vi "1.2.1-ParseYPR.vi"(10 "Serial Byte":u8) -> (1 "Yaw":i16, 2 "Heading (out)":T1)   [LabVIEW 2010]
doc: "This VI parses Yaw, Pitch, and Roll (YPR) data from the VectorNav. In response to a YPR Read Request, the VectorNav will reply in the form \"$VNYPR,XX,-XXX.XX,-XXX.XX,+XXX.XX*XX\" (where X is a digit from 0-9). This string is in the form \"$<command type>,<access ID>, <yaw>,<pitch>,<roll>\".\n\nThe VI first waits for a $, then checks to make sure it has read \"VNYPR,\" correctly, then adds up each of the XX values and saves them appropriately. Since it receives these values one byte at a time , it must do some simple fixed point math to make sure the appropriate decimal value is saved."
uses:
  1.2.1-ParseYPR.ctl
panel:
  in  "Heading (in)":T1 {"Yaw" format="%.42g"; "Pitch" format="%.42g"; "Roll" format="%.42g"}
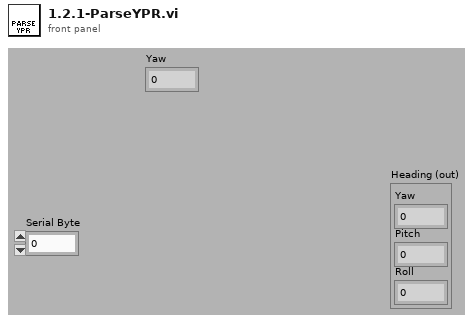
[diagram p1: front panel]
types:
  T1 = cluster{"Yaw":fxp<+/-,64,32>, "Pitch":fxp<+/-,64,32>, "Roll":fxp<+/-,64,32>}
  T2 = typedef "1.2.1-ParseYPR.ctl" = enum16{"Wait for $", "Check VNYPR", "Read numbers"}
  T3 = enum16{"Initialize", "Yaw", "Pitch", "Roll", "Done"}
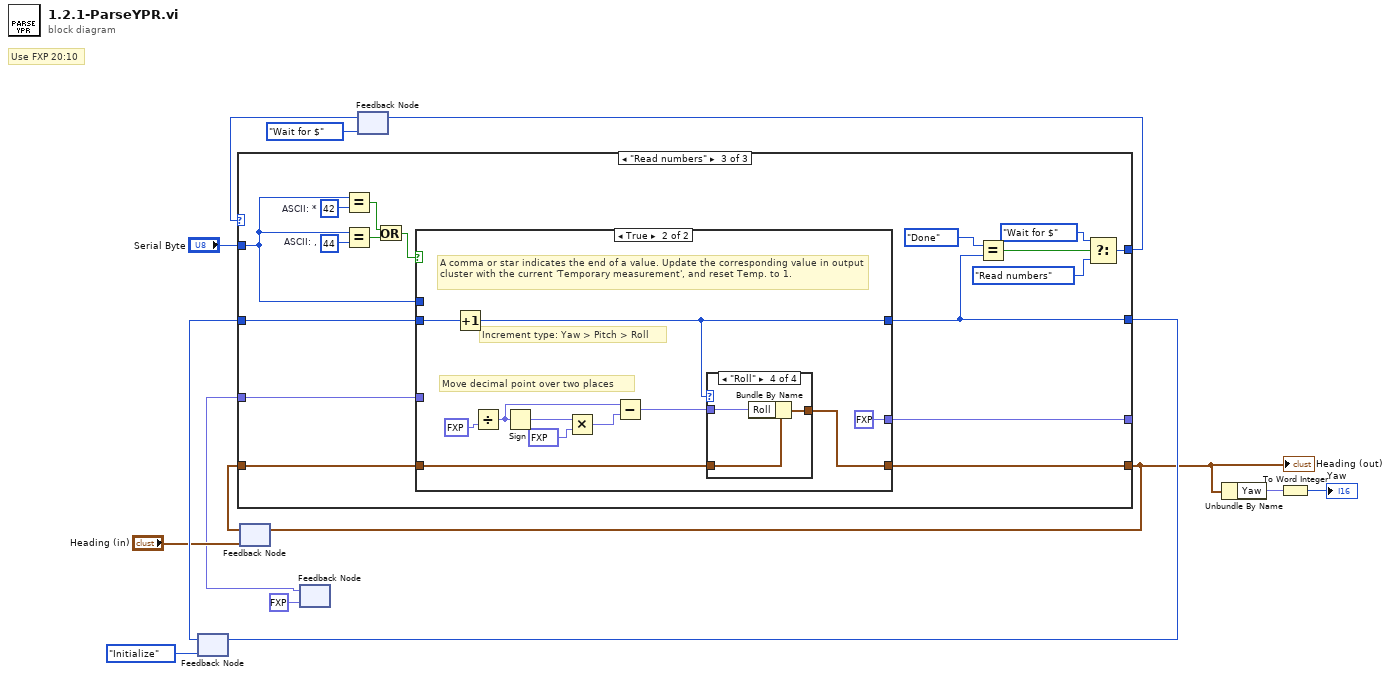
[diagram p0: block diagram]
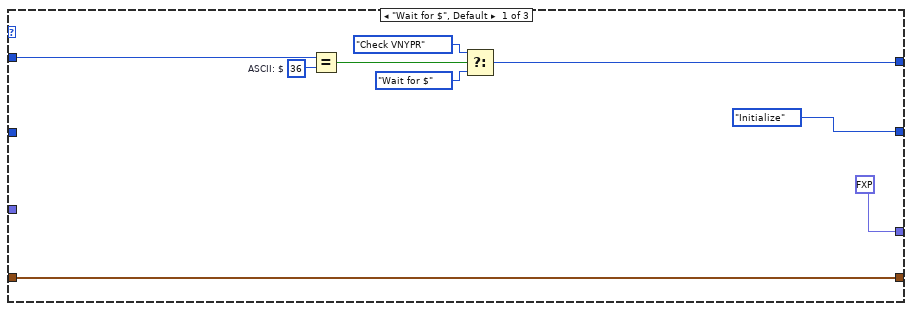
[diagram p2: hidden frame]
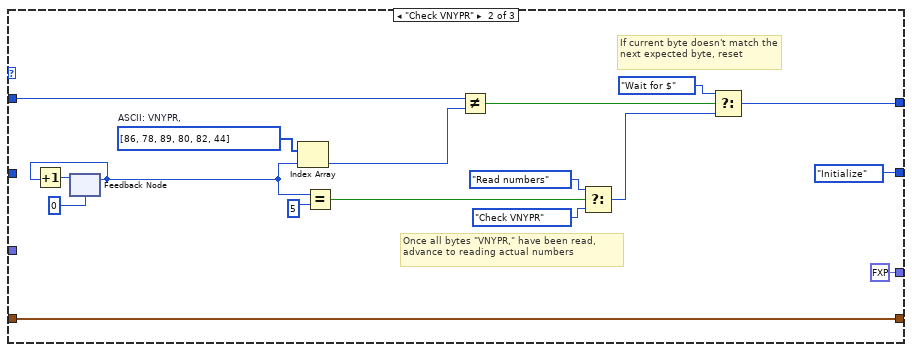
[diagram p3: hidden frame]
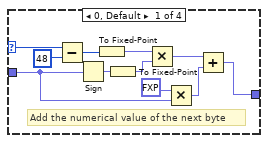
[diagram p5: hidden frame]
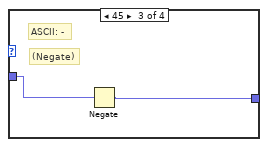
[diagram p6: hidden frame]
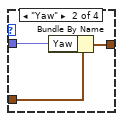
[diagram p9: hidden frame]
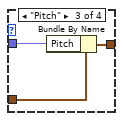
[diagram p10: hidden frame]
diagram:
  # "Use FXP 20:10"
  n1 = feedback #1(T3."Initialize" ("f")) -> (w8:T3)
  n2 = feedback #2("Heading (in)") -> (w11:T1)
  n3 = feedback #3(fxp<+/-,32,20> 1.0 ("Yaw")) -> (w1:fxp<+/-,32,20>)
  n4 = feedback-in #3() -> ()  [unwired: 1 out]
  n5 = feedback #4(1.2.1-ParseYPR."Wait for $" ("1.3.1-ParseYPR")) -> (w12:T2)
  n6 = case shown="\"Read numbers\"" w12 {
    tunnel: [w20 w29 w45] -> w14
    tunnel: "Serial Byte" -> [w23 w36 w44]
    tunnel: [fxp<+/-,32,20> 1.0 ("Yaw") fxp<+/-,32,20> 1.0 ("Yaw") w46] -> _
    tunnel: [w19 w37 w55] -> w5
    tunnel: w11 -> [w19 w37 w56]
    tunnel: [T3."Initialize" ("f") T3."Initialize" ("f") w53] -> w9
    tunnel: w8 -> [_ _ w54]
    tunnel: w1 -> [_ _ w41]
    frame "Wait for $", Default {
      w22 = u8 36  # ASCII: $
      n7 = Equal?(x=w23, y=w22) -> (x = y?=w21:bool)
      n8 = Select(t=1.2.1-ParseYPR."Check VNYPR" ("1.3.1-ParseYPR"), s=w21, f=1.2.1-ParseYPR."Wait for $" ("1.3.1-ParseYPR")) -> (s? t:f=w20:T2)
    }
    frame "Check VNYPR" {
      w40 = u8[] [86, 78, 89, 80, 82, 44]  # ASCII: VNYPR,
      # "If current byte doesn't match the next expected byte, reset"
      # "Once all bytes \"VNYPR,\" have been read, advance to reading actual numbers"
      n9 = feedback #5(0 ("Serial Byte")) -> (w24:i32)
      n10 = Increment(x=w24) -> (x+1=w25:i32)
      n11 = feedback-in #5(w25) -> ()
      n12 = Index Array(array=w40, index=w24) -> (element=w39:u8)
      n13 = Equal?(x=w24, y=5) -> (x = y?=w34:bool)
      n14 = Not Equal?(x=w36, y=w39) -> (x != y?=w38:bool)
      n15 = Select(t=1.2.1-ParseYPR."Read numbers" ("1.3.1-ParseYPR"), s=w34, f=1.2.1-ParseYPR."Check VNYPR" ("1.3.1-ParseYPR")) -> (s? t:f=w27:T2)
      n16 = Select(t=1.2.1-ParseYPR."Wait for $" ("1.3.1-ParseYPR"), s=w38, f=w27) -> (s? t:f=w29:T2)
    }
    frame "Read numbers" {
      w50 = u8 42  # ASCII: *
      w57 = u8 44  # ASCII: ,
      n17 = Equal?(x=w44, y=w50) -> (x = y?=w48:bool)
      n18 = Equal?(x=w44, y=w57) -> (x = y?=w49:bool)
      n19 = Or(x=w48, y=w49) -> (x .or. y?=w47:bool)
      n20 = case shown="True" w47 {
        tunnel: w56 -> [w62 w88]
        tunnel: [w62 w87] -> w55
        tunnel: [w61 w85] -> w53
        tunnel: w54 -> [w61 w86]
        tunnel: [w58 fxp<+/-,32,20> 1.0 ("Yaw")] -> w46
        tunnel: w44 -> [w60 _]
        tunnel: w41 -> [w59 _]
        frame False {
          # "Update current 'Temporary measurement'."
          n21 = case shown="43" w60 {
            selector: w60 -> [w72 _ _ _]
            tunnel: [w70 w74 w75 w77] -> w58
            tunnel: w59 -> [w64 w74 w76 w77]
            frame 0, Default {
              # "Add the numerical value of the next byte"
              n22 = Subtract(x=w72, y=u8 48) -> (x-y=w68:u8)
              n23 = Sign(1:w64) -> (0:w67:fxp<+/-,2,2>)
              n24 = To Fixed-Point(number=w68) -> (fixed-point=w66:fxp<+/-,32,20>)  [unwired: 1 in]
              n25 = To Fixed-Point(number=w67) -> (fixed-point=w65:fxp<+/-,32,20>)  [unwired: 1 in]
              n26 = Multiply(x=w66, y=w65) -> (x*y=w63:fxp<+/-,32,20>)
              n27 = Multiply(x=fxp<+/-,20,10> 10.0 ("Yaw"), y=w64) -> (x*y=w73:fxp<+/-,52,30>)
              n28 = Add(x=w63, y=w73) -> (x+y=w70:fxp<+/-,32,20>)
            }
            frame 43 {
              # "ASCII: +"
            }
            frame 45 {
              # "(Negate)"
              # "ASCII: -"
              n29 = Negate(x=w76) -> (-x=w75:fxp<+/-,33,21>)
            }
            frame 46 {
              # "(Ignore decimal for now)"
              # "ASCII: ."
            }
          }
        }
        frame True {
          # "Increment type: Yaw > Pitch > Roll"
          # "Move decimal point over two places"
          # "A comma or star indicates the end of a value. Update the corresponding value in output cluster with the current 'Temporary measurement', and reset Temp. to 1."
          n30 = Increment(x=w86) -> (x+1=w85:T3)
          n31 = Divide(y=fxp<+/-,32,20> 100.0 ("Yaw")) -> (x/y=w83:fxp<+/-,64,33>)  [unwired: 1 in]
          n32 = Sign(1:w83) -> (0:w81:fxp<+/-,2,2>)
          n33 = Multiply(x=w81, y=fxp<+/-,32,20> 1000.0 ("Yaw")) -> (x*y=w82:fxp<+/-,33,21>)
          n34 = Subtract(x=w83, y=w82) -> (x-y=w84:fxp<+/-,64,34>)
          n35 = case shown="\"Roll\"" w85 {
            tunnel: [w89 w92 w95 w98] -> w87
            tunnel: w88 -> [w89 w91 w94 w97]
            tunnel: w84 -> [_ w90 w93 w96]
            frame "Initialize", Default {
            }
            frame "Yaw" {
              n36 = Bundle By Name(cluster=w91, "Yaw"=w90) -> (w92:T1)
            }
            frame "Pitch" {
              n37 = Bundle By Name(cluster=w94, "Pitch"=w93) -> (w95:T1)
            }
            frame "Roll" {
              n38 = Bundle By Name(cluster=w97, "Roll"=w96) -> (w98:T1)
            }
          }
        }
      }
      n39 = Equal?(x=T3."Done", y=w53) -> (x = y?=w51:bool)
      n40 = Select(t=1.2.1-ParseYPR."Wait for $" ("1.3.1-ParseYPR"), s=w51, f=1.2.1-ParseYPR."Read numbers" ("1.3.1-ParseYPR")) -> (s? t:f=w45:T2)
    }
  }
  "Heading (out)" <- w5
  n41 = feedback-in #1(w9) -> ()
  n42 = feedback-in #2(w5) -> ()
  n43 = feedback-in #4(w14) -> ()
  n44 = Unbundle By Name(w5) -> ("Yaw"=w4:fxp<+/-,64,32>)
  n45 = To Word Integer(number=w4) -> (16bit integer=→"Yaw":i16)
